vi "Test Tag Read WAV.vi"(8 "error in (no error)":errorcluster) -> (0 "error out":errorcluster, 3 "Pass?":bool)   [LabVIEW 2020]
uses:
  G-Audio/G-Audio.lvlib
  G-Audio/Audio Files/Polymorphic VIs/Get Audio File Tags (Path).vi
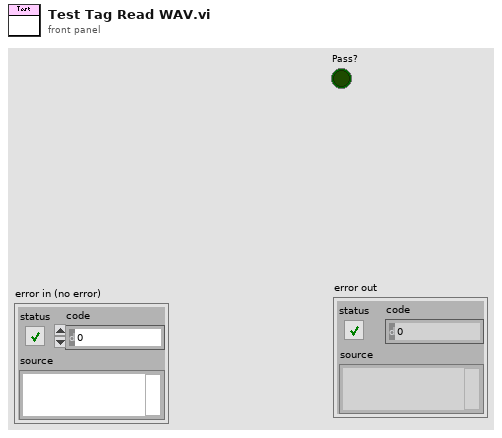
[diagram p1: front panel]
types:
  T1 = typedef "G-Audio.lvlib/Audio File Tag.ctl" = cluster{"Field":string, "Value":string}
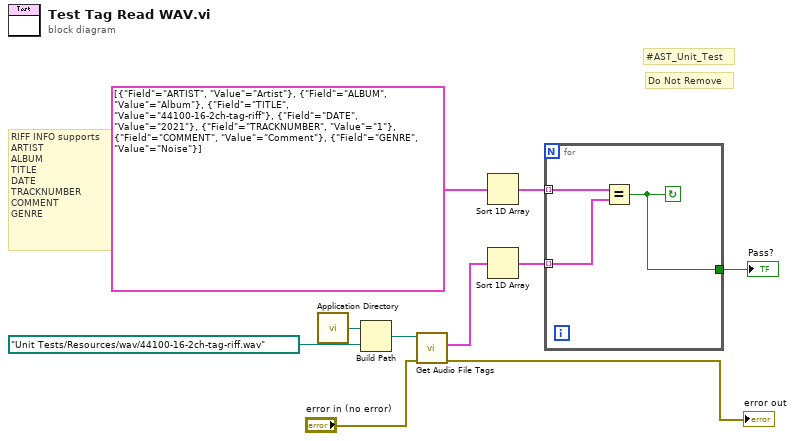
[diagram p0: block diagram]
diagram:
  # "RIFF INFO supports\nARTIST\nALBUM\nTITLE\nDATE\nTRACKNUMBER\nCOMMENT\nGENRE"
  # "Do Not Remove"
  # "#AST_Unit_Test"
  n1 = call <vilib>:"Application Directory.vi"() -> ("Application Directory"=w10:path)
  n2 = Build Path(base path=w10, name or relative path=path "Unit Tests/Resources/wav/44100-16-2ch-tag-riff.wav" ("Path")) -> (appended path=w8:path)
  n3 = call-poly "Get Audio File Tags.vi"("error in (no error)"="error in (no error)", "Path In"=w8) -> ("error out"=→"error out":errorcluster, "Tags"=w5:T1[])  [unwired: 7 in, 1 out]
  n4 = Sort 1D Array(array=cluster{"Field":string, "Value":string}[] [{"Field"="ARTIST", "Value"="Artist"}, {"Field"="ALBUM", "Value"="Album"}, {"Field"="TITLE", "Value"="44100-16-2ch-tag-riff"}, {"Field"="DATE", "Value"="2021"}, {"Field"="TRACKNUMBER", "Value"="1"}, {"Field"="COMMENT", "Value"="Comment"}, {"Field"="GENRE", "Value"="Noise"}]) -> (sorted array=w3:cluster{"Field":string, "Value":string}[])
  n5 = Sort 1D Array(array=w5) -> (sorted array=w4:T1[])
  n6 = for {
    tunnel: w4 -> [w11] mode=indexing
    tunnel: w3 -> [w13] mode=indexing
    tunnel: [w12] -> w1
    stop <- w12 continue-if-true
    n7 = Equal?(x=w13, y=w11) -> (x = y?=w12:bool)
  }
  "Pass?" <- w1
